vi "read serial number.vi"(8 "error in":errorcluster, 11 "device in":refnum<class "Device.lvclass">) -> (0 "error out":errorcluster, 2 "serial number":string, 3 "device out":refnum<class "Device.lvclass">)   [LabVIEW 2013, in "SMI.lvlib" / "Device.lvclass"]
uses:
  Device.lvclass
  Device.lvclass/Device.ctl
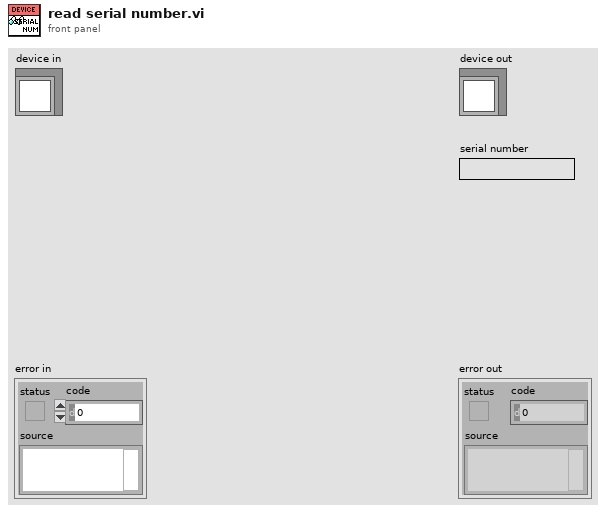
[diagram p1: front panel]
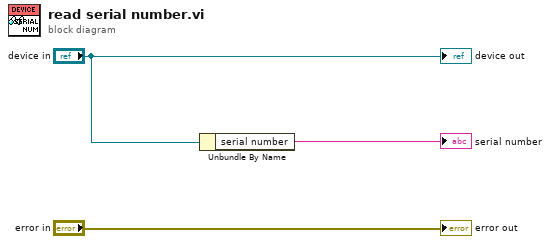
[diagram p0: block diagram]
diagram:
  n1 = Unbundle By Name("device in") -> ("serial number"=→"serial number":string)
  "error out" <- "error in"
  "device out" <- "device in"
